vi "tcp_send.vi"() -> ()   [LabVIEW 2018]
panel:
  in  "Server Closed":string="The server VI closed the connection."
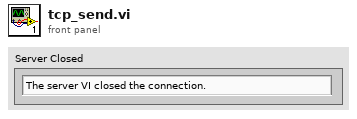
[diagram p1: front panel]
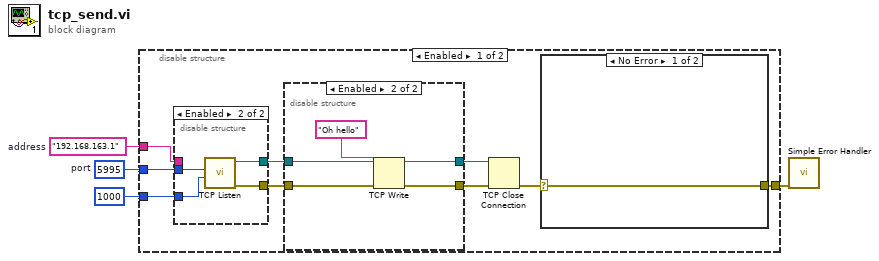
[diagram p0: block diagram]
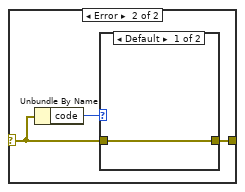
[diagram p2: hidden frame]
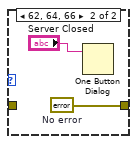
[diagram p3: hidden frame]
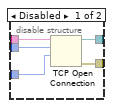
[diagram p4: hidden frame]
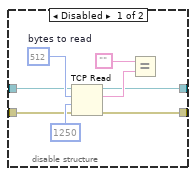
[diagram p5: hidden frame]
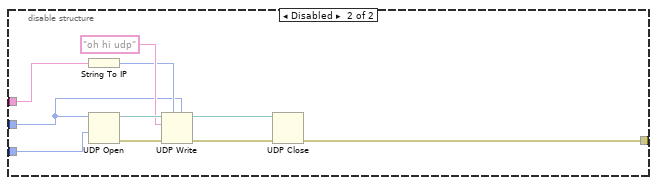
[diagram p6: hidden frame]
diagram:
  w3 = u16 5995  # port
  w4 = "192.168.163.1"  # address
  n1 = disable-structure shown="Enabled" {
    disable-tunnel: w4 -> [w13 w47]
    disable-tunnel: w3 -> [w12 w46]
    disable-tunnel: [w6 w43] -> w2
    disable-tunnel: 1000 ("timeout ms (60000)") -> [w5 w52]
    frame Enabled {
      n2 = disable-structure shown="Enabled" {
        disable-tunnel: [w25 w28] -> w11
        disable-tunnel: [w24 w29] -> w10
        disable-tunnel: w13 -> [w23 _]
        disable-tunnel: w12 -> [w21 w27]
        disable-tunnel: w5 -> [w22 w26]
        frame Disabled {
          n3 = TCP Open Connection(address=w23, remote port or service name=w21, timeout ms (60000)=w22) -> (connection ID=w25:refnum<k5>, error out=w24:errorcluster)  [unwired: 2 in]
        }
        frame Enabled {
          n4 = call <vilib>:"TCP Listen.vi"("timeout ms (wait forever: -1)"=w26, "port"=w27) -> ("error out"=w29:errorcluster, "connection ID"=w28:refnum<k5>)  [unwired: 5 in, 3 out]
        }
      }
      n5 = disable-structure shown="Enabled" {
        disable-tunnel: w11 -> [w33 w38]
        disable-tunnel: w10 -> [w32 w39]
        disable-tunnel: [w30 w41] -> w9
        disable-tunnel: [w31 w40] -> w8
        frame Disabled {
          w37 = 512  # bytes to read
          n6 = TCP Read(connection ID=w33, bytes to read=w37, error in (no error)=w32, 9:1250 ("timeout ms (25000)")) -> (connection ID out=w31:refnum<k5>, data out=w34:string, error out=w30:errorcluster)  [unwired: 1 in]
          n7 = Equal?(x="", y=w34) -> ()  [unwired: 1 out]
        }
        frame Enabled {
          n8 = TCP Write(connection ID=w38, data in="Oh hello", error in (no error)=w39) -> (connection ID out=w40:refnum<k5>, error out=w41:errorcluster)  [unwired: 2 out]
        }
      }
      n9 = TCP Close Connection(connection ID=w8, error in (no error)=w9) -> (error out=w7:errorcluster)  [unwired: 1 in, 1 out]
      n10 = case shown="No Error" w7 {
        selector: w7 -> [w14 w16]
        tunnel: [w14 w15] -> w6
        frame No Error {
        }
        frame Error {
          n11 = Unbundle By Name(w16) -> ("code"=w17:i32)
          n12 = case shown="Default" w17 {
            tunnel: w16 -> [w18 _]
            tunnel: [w18 w20] -> w15
            frame Default {
            }
            frame 62, 64, 66 {
              w20 = errorcluster {"status"=FALSE, "code"=0, "source"=""}  # No error
              n13 = One Button Dialog(message="Server Closed") -> ()  [unwired: 1 in, 1 out]
            }
          }
        }
      }
    }
    frame Disabled {
      n14 = String To IP(1:w47) -> (0:w48:u32)
      n15 = UDP Open(9:w52, 11:w46) -> (port=w51:refnum<k16>, 0:w50:errorcluster)  [unwired: 3 in, 1 out]
      n16 = UDP Write(address=w48, port or service name=w46, connection ID=w51, data in="oh hi udp" ("address"), 8:w50) -> (error out=w44:errorcluster, 3:w45:refnum<k16>)  [unwired: 1 in]
      n17 = UDP Close(connection ID=w45, 8:w44) -> (error out=w43:errorcluster)  [unwired: 1 out]
    }
  }
  n18 = call <vilib>:"Simple Error Handler.vi"("error in (no error)"=w2) -> ()  [unwired: 4 in, 5 out]
